vi "OFDM-SIM子载波部分.vi"(0 "输入前53个序列":cdb[](array[numeric]), 1 "error in":errorcluster caption="error in (no error)") -> (2 "总比特数":i32, 3 "错误比特数":i32, 4 "error out":errorcluster)   [LabVIEW 2018]
uses:
  <vilib>/addons/Modulation/Digital/General/MT Generate QAM System Parameters(M).vi
  <vilib>/addons/Modulation/Digital/General/MT Map QAM Symbols to Bits.vi
  <vilib>/addons/Modulation/niDMT.lvlib
panel:
  out "激活子载波输出的比特":i8[](array[numeric]) caption="output bit stream"
  out "激活子载波的索引":i32[](array[numeric])
  out "大小 2":i32
  out "星座图":cdb[](graph)
  out "输出符号":cdb[](array[numeric])
  out "除去导频后的符号":cdb[](array[numeric])
  out "除去导频后的信道参数":cdb[](array[numeric])
  out "插入的导频序列":cdb[](array[numeric])
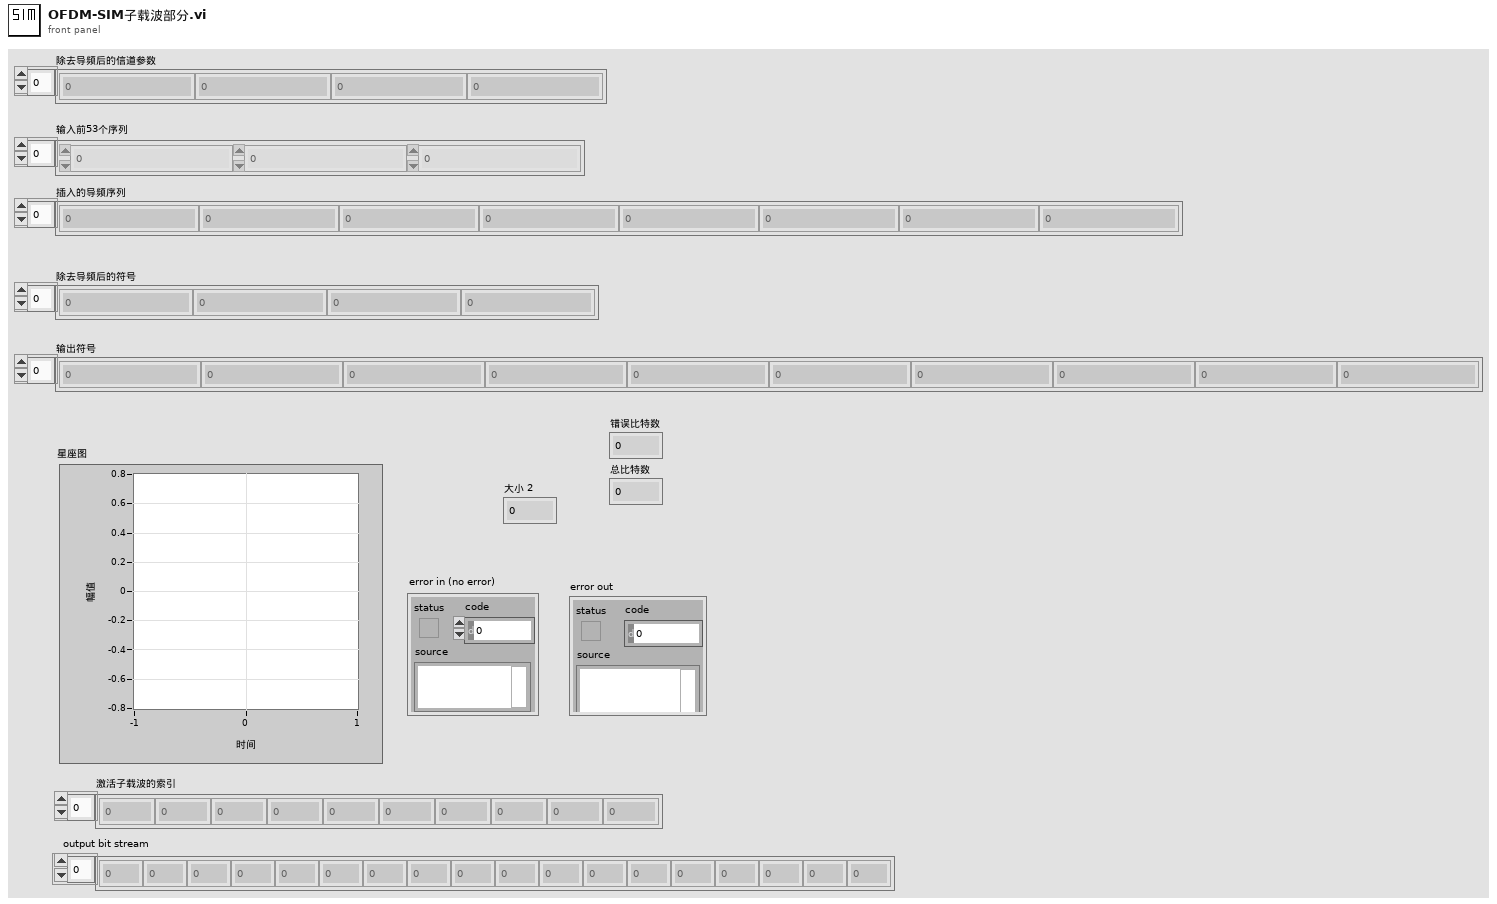
[diagram p1: front panel]
types:
  T1 = cluster{"samples per symbol (16)":i32, "symbol map":cdb[]}
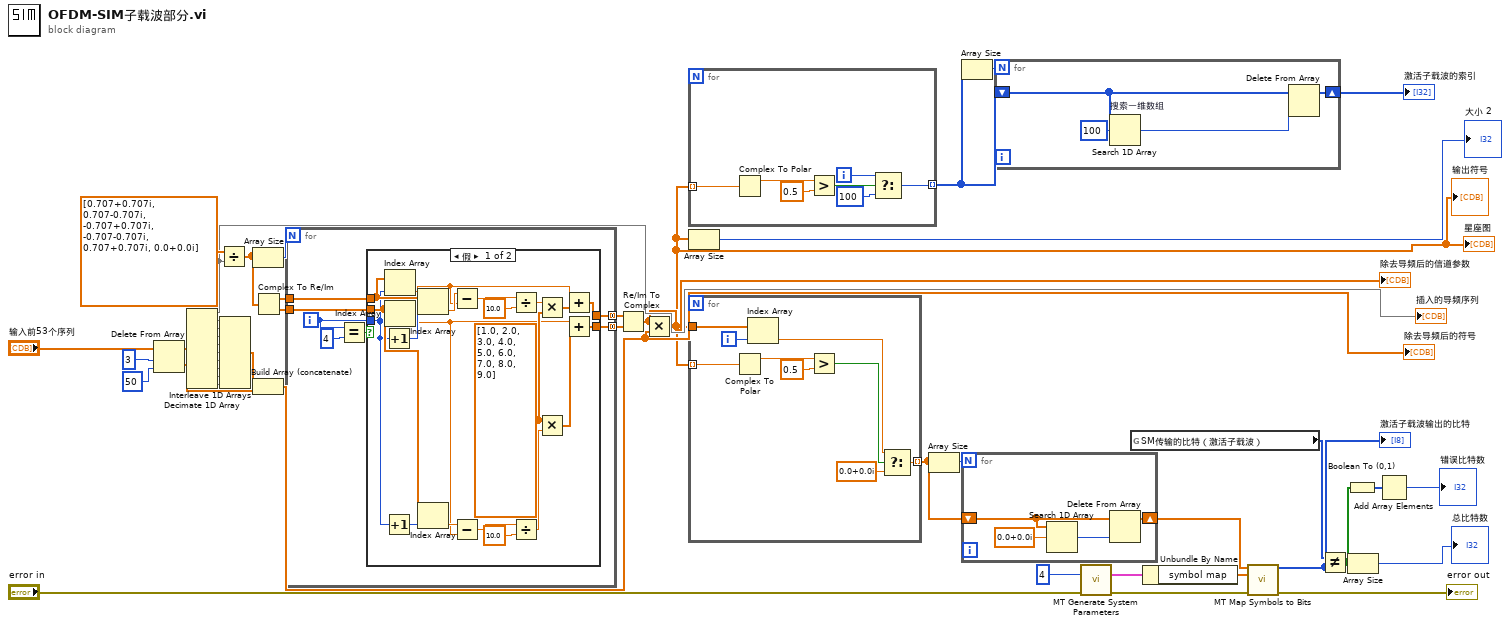
[diagram p0: block diagram]
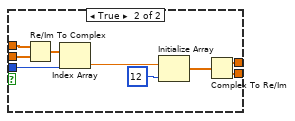
[diagram p2: hidden frame]
diagram:
  n1 = Delete From Array(array="输入前53个序列", length=3 ("长度"), index=50 ("索引")) -> (deleted portion=w25:cdb[], array with subset deleted=w26:cdb[])
  n2 = Decimate 1D Array(w26) -> (w23:cdb[], w30:cdb[], w31:cdb[], w32:cdb[], w33:cdb[], w34:cdb[], w35:cdb[], w36:cdb[], w37:cdb[], w38:cdb[])
  "插入的导频序列" <- w23
  n3 = Divide(x=cdb[] [0.707+0.707i, 0.707-0.707i, -0.707+0.707i, -0.707-0.707i, 0.707+0.707i, 0.0+0.0i] ("数组"), y=w23) -> (x/y=w43:cdb[])
  n4 = Interleave 1D Arrays(w30, w31, w32, w33, w34, w35, w36, w37, w38) -> (w24:cdb[])
  n5 = Array Size(array=w43) -> (size(s)=w44:i32)
  n6 = Build Array (concatenate)(w24, w25) -> (w22:cdb[])
  "除去导频后的符号" <- w22
  n7 = Complex To Re/Im(x + iy=w43) -> (x=w42:dbl[], y=w41:dbl[])
  n8 = for {
    N: w44 -> [_]
    tunnel: w42 -> [w51]
    tunnel: w41 -> [w49]
    tunnel: [w47] -> w40 mode=concatenating
    tunnel: [w46] -> w39 mode=concatenating
    i -> [w48]
    n9 = Equal?(x=w48, y=4) -> (x = y?=w50:bool)
    n10 = case shown="假" w50 {
      tunnel: w51 -> [w72 w81]
      tunnel: w49 -> [w70 w80]
      tunnel: [w55 w76] -> w47
      tunnel: [w54 w75] -> w46
      tunnel: w48 -> [w53 w73]
      frame False {
        w59 = dbl[] [1.0, 2.0, 3.0, 4.0, 5.0, 6.0, 7.0, 8.0, 9.0] ("y")
        n11 = Increment(x=w53) -> (x+1=w71:i32)
        n12 = Increment(x=w53) -> (x+1=w69:i32)
        n13 = Index Array(array=w72, index=w53) -> (element=w64:dbl)
        n14 = Index Array(array=w70, index=w53) -> (element=w57:dbl)
        n15 = Index Array(array=w72, index=w71) -> (element=w68:dbl)
        n16 = Index Array(array=w70, index=w69) -> (element=w63:dbl)
        n17 = Subtract(x=w68, y=w64) -> (x-y=w67:dbl)
        n18 = Subtract(x=w63, y=w57) -> (x-y=w62:dbl)
        n19 = Divide(x=w67, y=10.0) -> (x/y=w66:dbl)
        n20 = Divide(x=w62, y=10.0) -> (x/y=w60:dbl)
        n21 = Multiply(x=w66, y=w59) -> (x*y=w65:dbl[])
        n22 = Multiply(x=w59, y=w60) -> (x*y=w56:dbl[])
        n23 = Add(x=w64, y=w65) -> (x+y=w55:dbl[])
        n24 = Add(x=w57, y=w56) -> (x+y=w54:dbl[])
      }
      frame True {
        n25 = Re/Im To Complex(1:w80, 2:w81) -> (0:w79:cdb[])
        n26 = Index Array(array=w79, index=w73) -> (element=w78:cdb)
        n27 = Initialize Array(w78, 12 ("维数大小")) -> (w77:cdb[])
        n28 = Complex To Re/Im(x + iy=w77) -> (x=w76:dbl[], y=w75:dbl[])
      }
    }
  }
  n29 = Re/Im To Complex(1:w39, 2:w40) -> (0:w21:cdb[])
  "除去导频后的信道参数" <- w21
  n30 = Multiply(x=w21, y=w22) -> (x*y=w11:cdb[])
  "输出符号" <- w11
  "星座图" <- w11
  n31 = for {
    tunnel: w11 -> [w88] mode=indexing
    tunnel: [w83] -> w14 mode=indexing
    i -> [w84]
    n32 = Complex To Polar(r * e^(i*theta)=w88) -> (r=w87:dbl)  [unwired: 1 out]
    n33 = Greater?(x=w87, y=0.5) -> (0:w85:bool)
    n34 = Select(t=w84, s=w85, f=100) -> (s? t:f=w83:i32)
  }
  n35 = Array Size(array=w11) -> (size(s)=→"大小 2":i32)
  n36 = for {
    tunnel: w11 -> [w95] mode=indexing
    tunnel: w11 -> [w93]
    tunnel: [w89] -> w9 mode=indexing
    i -> [w92]
    n37 = Complex To Polar(r * e^(i*theta)=w95) -> (r=w97:dbl)  [unwired: 1 out]
    n38 = Index Array(array=w93, index=w92) -> (element=w91:cdb)
    n39 = Greater?(x=w97, y=0.5) -> (0:w94:bool)
    n40 = Select(t=w91, s=w94, f=cdb 0.0+0.0i) -> (s? t:f=w89:cdb)
  }
  n41 = Array Size(array=w9) -> (size(s)=w10:i32)
  n42 = Array Size(array=w14) -> (size(s)=w13:i32)
  n43 = for {
    N: w10 -> [_]
    shift-right: [w100] -> w8
    shift-left: w9 -> [w99]
    n44 = Search 1D Array ("搜索一维数组")(1D array=w99, element=cdb 0.0+0.0i ("f")) -> (index of element=w98:i32)  [unwired: 1 in]
    n45 = Delete From Array(array=w99, index=w98) -> (array with subset deleted=w100:cdb[])  [unwired: 1 in, 1 out]
  }
  n46 = for {
    N: w13 -> [_]
    shift-right: [w102] -> w12
    shift-left: w14 -> [w104]
    n47 = Search 1D Array "搜索一维数组"(1D array=w104, element=100 ("元素")) -> (index of element=w103:i32)  [unwired: 1 in]
    n48 = Delete From Array(array=w104, index=w103) -> (array with subset deleted=w102:i32[])  [unwired: 1 in, 1 out]
  }
  "激活子载波的索引" <- w12
  n49 = call-poly <vilib>:"MT Generate System Parameters.vi"("M-QAM (16)"=4, "error in (no error)"="error in") -> ("QAM system parameters"=w20:T1, "error out"=w17:errorcluster)  [unwired: 11 in, 1 out]
  n50 = global read "SM传输的序列（激活子载波）.vi" "SM传输的比特（激活子载波）"() -> (w4:i32[])
  n51 = Unbundle By Name(w20) -> ("symbol map"=w19:cdb[])
  n52 = call-poly <vilib>:"MT Map Symbols to Bits.vi"("symbols"=w8, "symbol map"=w19, "error in (no error)"=w17) -> ("output bit stream"=w5:i8[], "error out"=→"error out":errorcluster)  [unwired: 11 in]
  "激活子载波输出的比特" <- w5
  n53 = Not Equal?(x=w4, y=w5) -> (x != y?=w6:bool[])
  n54 = Boolean To (0,1)(Boolean=w6) -> (0, 1=w7:i16[])
  n55 = Array Size(array=w6) -> (size(s)=→"总比特数":i32)
  n56 = Add Array Elements(numeric array=w7) -> (sum=→"错误比特数":i16)
